vi "Polynomial Second Derivitive.vi"(2 "CX^2":dbl, 3 "DX^3":dbl, 4 "EX^4":dbl, 5 "FX^5":dbl, 6 "X":dbl) -> (16 "Y":dbl)   [LabVIEW 2015]
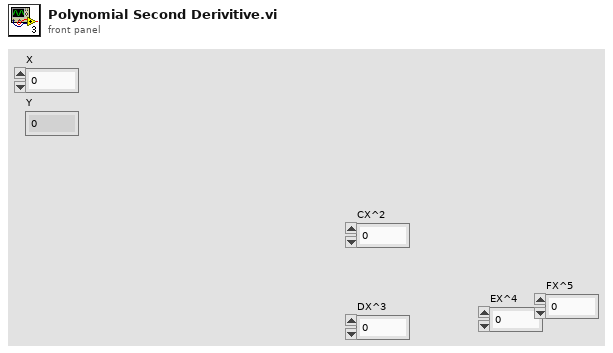
[diagram p1: front panel]
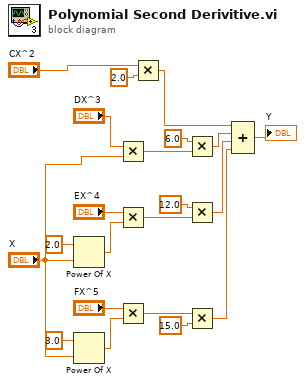
[diagram p0: block diagram]
diagram:
  n1 = Power Of X(1:"X", 2:2.0 ("y")) -> (0:w19:dbl)
  n2 = Power Of X(1:"X", 2:3.0 ("y")) -> (0:w16:dbl)
  n3 = Multiply(x="DX^3", y="X") -> (x*y=w14:dbl)
  n4 = Multiply(x="EX^4", y=w19) -> (x*y=w13:dbl)
  n5 = Multiply(x="FX^5", y=w16) -> (x*y=w12:dbl)
  n6 = Multiply(x="CX^2", y=2.0) -> (x*y=w10:dbl)
  n7 = Multiply(x=6.0, y=w14) -> (x*y=w8:dbl)
  n8 = Multiply(x=12.0, y=w13) -> (x*y=w6:dbl)
  n9 = Multiply(x=w12, y=15.0) -> (x*y=w4:dbl)
  n10 = Compound Arithmetic op=ADD(w10, w8, w6, w4) -> (→"Y":dbl)
